vi "configure update.vi"(4 "Username (\"\")":string, 5 "error in (no error)":errorcluster, 8 "POST (empty)":T1) -> (0 "error out":errorcluster, 3 "Updates":string)   [LabVIEW 2011]
uses:
  ITK EXT/utils/keyedarr.llb/Keyed Array.ctl
  ITK EXT/utils/strutil.llb/Case Matching.ctl
  server/server lib/Spartan CONFIG Global.vi
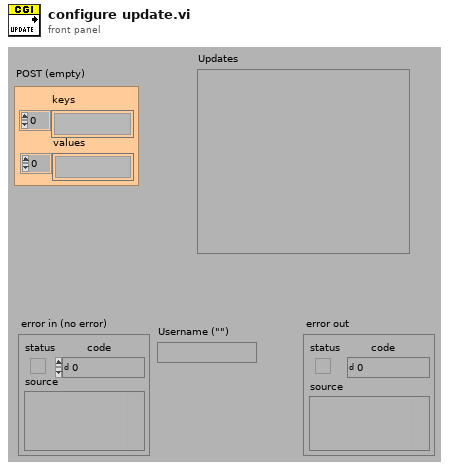
[diagram p1: front panel]
types:
  T1 = typedef "Keyed Array.ctl" = cluster{"keys":string[], "values":string[]}
  T2 = cluster{"key name":string, "key value":string, "default value":string}[]
  T3 = typedef "Case Matching.ctl" = enum16{"a != A", "a == A", "system"}
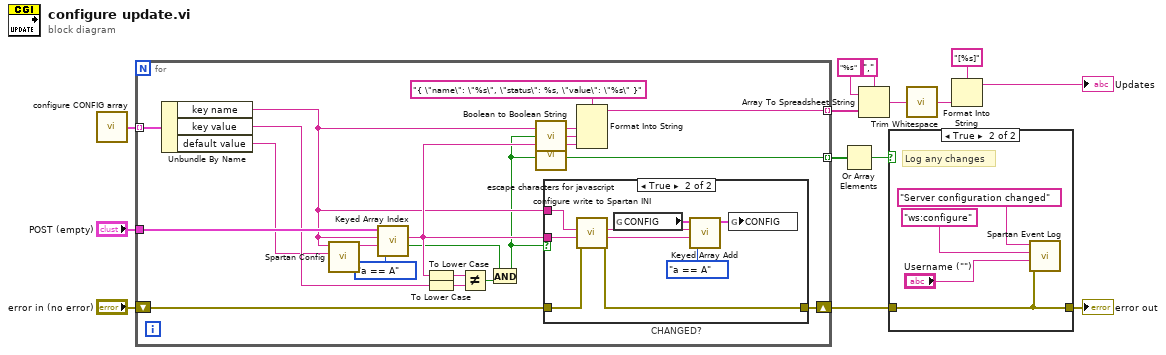
[diagram p0: block diagram]
diagram:
  n1 = call "configure CONFIG array.vi"() -> ("CONFIG"=w1:T2)
  n2 = for {
    shift-right: [w24] -> w7
    shift-left: "error in (no error)" -> [w23]
    tunnel: [w22] -> w5 mode=indexing
    tunnel: [w15] -> w6 mode=indexing
    tunnel: "POST (empty)" -> [w21]
    tunnel: w1 -> [w20] mode=indexing
    n3 = Unbundle By Name(w20) -> ("key name"=w19:string, "key value"=w18:string, "default value"=w17:string)
    n4 = call "Spartan Config.vi"("Default Value (\"\")"=w17, "Config Key (\"\")"=w19) -> ("Config Value"=w26:string)  [unwired: 7 in, 2 out]
    n5 = call "Keyed Array Index.vi"("case matching (sensitive)"=Case_Matching."a == A", "default value"=w26, "key"=w19, "array in"=w21) -> ("valid key"=w16:bool, "value"=w27:string)  [unwired: 2 out]
    n6 = To Lower Case(string=w27) -> (all lower case string=w32:string)
    n7 = To Lower Case(string=w18) -> (all lower case string=w33:string)
    n8 = Not Equal?(x=w32, y=w33) -> (x != y?=w25:bool)
    n9 = And(x=w16, y=w25) -> (x .and. y?=w15:bool)
    n10 = call "Boolean to Boolean String.vi"("Boolean"=w15) -> ("Boolean string"=w29:string)  [unwired: 1 in]
    n11 = call "escape characters for javascript.vi"("String (\"\")"=w27) -> ("escaped String"=w28:string)  [unwired: 4 out]
    n12 = case "CHANGED?" shown="True" w15 {
      tunnel: w23 -> [w34 w41]
      tunnel: [w34 w40] -> w24
      tunnel: w27 -> [_ w35]
      tunnel: w19 -> [_ w36]
      frame False {
      }
      frame True {
        n13 = call "configure write to Spartan INI.vi"("error in (no error)"=w41, "Value (\"\")"=w35, "Key (\"\")"=w36) -> ("error out"=w40:errorcluster)  [unwired: 8 in]
        n14 = global read "Spartan CONFIG Global.vi" "CONFIG"() -> (w38:T1)
        n15 = call "Keyed Array Add.vi"("case matching (sensitive)"=Case_Matching."a == A", "value"=w35, "key"=w36, "array in"=w38) -> ("array out"=w37:T1)  [unwired: 3 out]
        n16 = global write "Spartan CONFIG Global.vi" "CONFIG"(w37) -> ()
      }
    }
    n17 = Format Into String(format string="{ \"name\": \"%s\", \"status\": %s, \"value\": \"%s\" }", w19, w29, w28) -> (resulting string=w22:string)  [unwired: 2 in, 1 out]
  }
  n18 = Or Array Elements(Boolean array=w6) -> (logical OR=w4:bool)
  n19 = Array To Spreadsheet String(delimiter (Tab)=",", array=w5, 3:"%s") -> (spreadsheet string=w13:string)
  n20 = case shown="True" w4 {
    tunnel: w7 -> [w42 w43]
    tunnel: [w42 w43] -> w12
    frame False {
    }
    frame True {
      # "Log any changes"
      n21 = call "Spartan Event Log.vi"("error in (no error)"=w43, "username (\"\")"="Username (\"\")", "module (\"\")"="ws:configure" ("module (\"\")"), "message (\"\")"="Server configuration changed" ("virtual path")) -> ()  [unwired: 4 in, 1 out]
    }
  }
  "error out" <- w12
  n22 = call <vilib>:"Trim Whitespace.vi"("string"=w13) -> ("trimmed string"=w9:string)  [unwired: 1 in]
  n23 = Format Into String(format string="[%s]", w9) -> (resulting string=→"Updates":string)  [unwired: 2 in, 1 out]
